vi "Reshape data.vi"(9 "Logging queue element in":T1={"Imaging Protocol"=enum."Live Imaging", "Number of Trials"=0, "Frame Size"=512, "# Averaged frames"=0, "Dwell time (us)"=0.0, "Index of Z-plane"=0, "Timelapse?"=FALSE, "Logging process is active"=FALSE, "Speed logging enabled"=FALSE, "tdms file ref"=refnum, "path"=path "", "Trial Number"=0, "Expected # points acquired"=FALSE, "Manually stopped"=FALSE, "Ch0 data"=[], "Ch1 data"=[], "Ref Data"=[], "Last trial"=FALSE, "Ref Dwell time (us)"=0.0, "# Ref Averaged frames"=0, "Ref X Length"=0, "Ref Y Length"=0, "Points acquired"={"Ch0 last trial"=0, "Ch1 last trial"=0, "All trials"=0}} {"Ref Dwell time (us)" format="%#.6g"; "Frame Size" items=["100X100"=100, "128X128"=128, "200X200"=200, "256X256"=256, "512X512"=512, "1024x1024"=1024, "2048x2048"=2048]; "Dwell time (us)" format="%#.6g"}, 11 "Data":T5) -> (0 "Ch1 has data":bool, 1 "Ch0 has data":bool, 2 "Ch1-Green":i16[][](array[numeric]), 3 "Ch0-Red":i16[][](array[numeric]))   [LabVIEW 2017]
uses:
  Typedefs/Frame data dual cluster.ctl
  Typedefs/Logging queue element.ctl
  Typedefs/Imaging Protocols enum.ctl
  Typedefs/Frame Size.ctl
  Typedefs/Acquired points count.ctl
panel:
  # "SUBROUTINE VI"
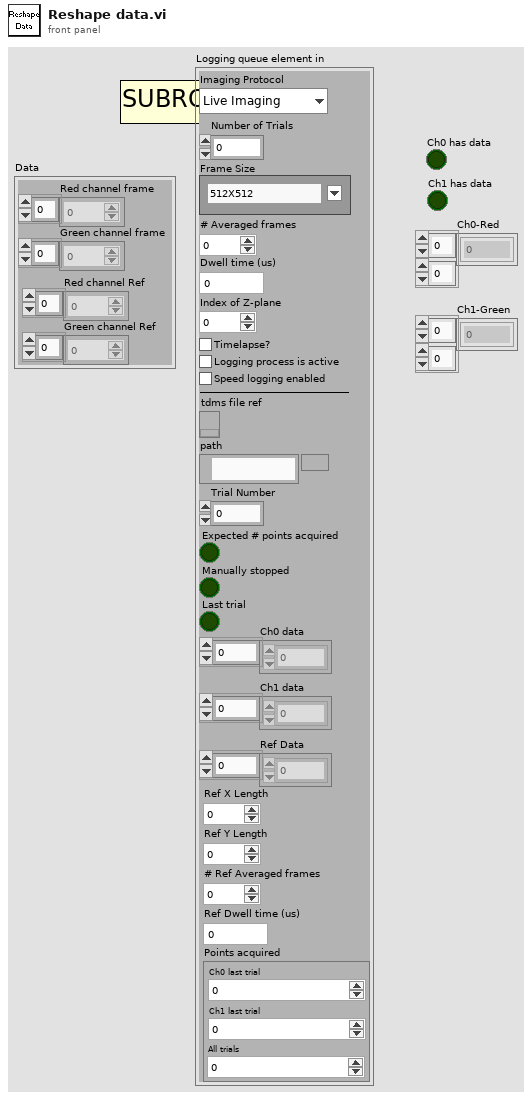
[diagram p1: front panel]
types:
  T1 = typedef "Logging queue element.ctl" = cluster{"Imaging Protocol":T2, "Number of Trials":u16, "Frame Size":T3, "# Averaged frames":u16, "Dwell time (us)":dbl, "Index of Z-plane":i32, "Timelapse?":bool, "Logging process is active":bool, "Speed logging enabled":bool, "tdms file ref":refnum<k34>, "path":path, "Trial Number":i32, "Expected # points acquired":bool, "Manually stopped":bool, "Ch0 data":u32[], "Ch1 data":u32[], "Ref Data":u32[], "Last trial":bool, "Ref Dwell time (us)":dbl, "# Ref Averaged frames":u16, "Ref X Length":u16, "Ref Y Length":u16, "Points acquired":T4}
  T2 = typedef "Imaging Protocols enum.ctl" = enum16{"AOL Z-Stack", "Motor Z Stack", "Functional Acquisition", "Single Plane Acquisition", "Volume Acquisition", "Live Imaging", "Live Plane Imaging", "Live Volume Imaging"}
  T3 = typedef "Frame Size.ctl" = u16
  T4 = typedef "Acquired points count.ctl" = cluster{"Ch0 last trial":u64, "Ch1 last trial":u64, "All trials":u64}
  T5 = typedef "Frame data dual cluster.ctl" = cluster{"Red channel frame":dbl[], "Green channel frame":dbl[], "Red channel Ref":dbl[], "Green channel Ref":dbl[]}
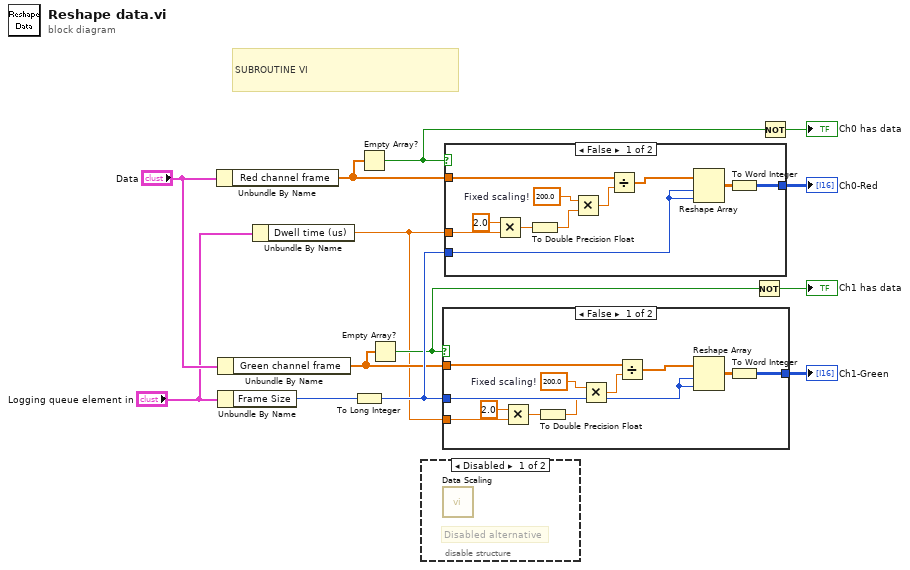
[diagram p0: block diagram]
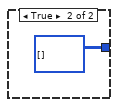
[diagram p3: hidden frame]
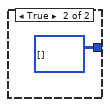
[diagram p4: hidden frame]
diagram:
  # "SUBROUTINE VI"
  n1 = Unbundle By Name("Data") -> ("Red channel frame"=w8:dbl[])
  n2 = Unbundle By Name("Data") -> ("Green channel frame"=w2:dbl[])
  n3 = Unbundle By Name("Logging queue element in") -> ("Frame Size"=w9:T3)
  n4 = Unbundle By Name("Logging queue element in") -> ("Dwell time (us)"=w1:dbl)
  n5 = To Long Integer(number=w9) -> (32bit integer=w11:i32)
  n6 = Empty Array?(array=w8) -> (empty?=w7:bool)
  n7 = Empty Array?(array=w2) -> (empty?=w6:bool)
  n8 = disable-structure shown="Disabled" {
    frame Disabled {
      # "Disabled alternative"
      n9 = call "Data Scaling.vi"() -> ()  [unwired: 14 in, 2 out]
    }
    frame Enabled {
    }
  }
  n10 = case shown="False" w6 {
    tunnel: w2 -> [w17 _]
    tunnel: [w24 i16[][] []] -> w13
    tunnel: w11 -> [w23 _]
    tunnel: w1 -> [w15 _]
    frame False {
      w14 = 200.0  # Fixed scaling!
      n11 = Multiply(x=2.0, y=w15) -> (x*y=w20:dbl)
      n12 = To Double Precision Float(number=w20) -> (double precision float=w19:dbl)
      n13 = Multiply(x=w14, y=w19) -> (x*y=w18:dbl)
      n14 = Divide(x=w17, y=w18) -> (x/y=w16:dbl[])
      n15 = Reshape Array(w16, w23, w23) -> (w22:dbl[][])
      n16 = To Word Integer(number=w22) -> (16bit integer=w24:i16[][])
    }
    frame True {
    }
  }
  "Ch1-Green" <- w13
  n17 = case shown="False" w7 {
    tunnel: [w36 i16[][] []] -> w12
    tunnel: w11 -> [w35 _]
    tunnel: w8 -> [w29 _]
    tunnel: w1 -> [w27 _]
    frame False {
      w26 = 200.0  # Fixed scaling!
      n18 = Multiply(x=2.0, y=w27) -> (x*y=w31:dbl)
      n19 = To Double Precision Float(number=w31) -> (double precision float=w32:dbl)
      n20 = Multiply(x=w26, y=w32) -> (x*y=w33:dbl)
      n21 = Divide(x=w29, y=w33) -> (x/y=w28:dbl[])
      n22 = Reshape Array(w28, w35, w35) -> (w34:dbl[][])
      n23 = To Word Integer(number=w34) -> (16bit integer=w36:i16[][])
    }
    frame True {
    }
  }
  "Ch0-Red" <- w12
  n24 = Not(x=w6) -> (.not. x?=→"Ch1 has data":bool)
  n25 = Not(x=w7) -> (.not. x?=→"Ch0 has data":bool)
